vi "analog2digital_wf_array.vi"(8 "error in (no error)":errorcluster, 11 "analog waveform":waveform(dbl)) -> (0 "error out":errorcluster, 1 "full-scale range (out)":dbl, 2 "resolution (out)":i32=16, 3 "digital array":digitalwaveform[](array[waveform]))   [LabVIEW 2015]
uses:
  <vilib>/Waveform/DWDTOps.llb/DWDT Analog to Digital.vi
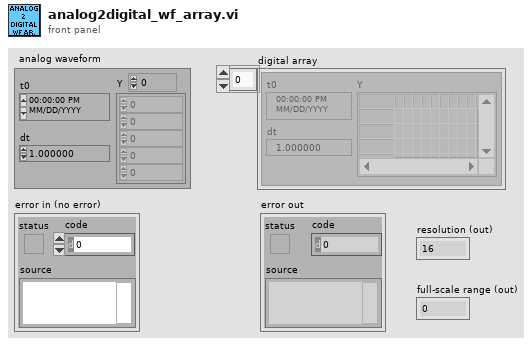
[diagram p1: front panel]
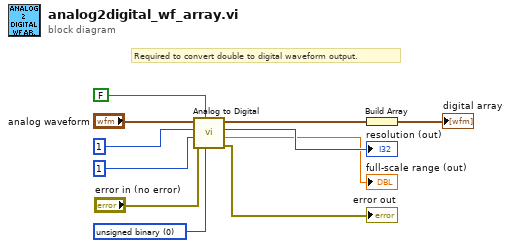
[diagram p0: block diagram]
diagram:
  w6 = u16 0 items=["unsigned binary", "offset binary", "2's complement"] ("data format (offset binary)")
  # "Required to convert double to digital waveform output."
  n1 = call-poly <vilib>:"Analog to Digital.vi"("data format (offset binary)"=w6, "compress digital (T)"=FALSE, "error in (no error)"="error in (no error)", "full-scale range (pk-pk)"=1 ("resolution (16 bit)"), "resolution (16 bit)"=1, "analog waveform"="analog waveform") -> ("error out"=→"error out":errorcluster, "full-scale range (out)"=→"full-scale range (out)":dbl, "resolution (out)"=→"resolution (out)":i32, "digital waveform"=w10:digitalwaveform)  [unwired: 2 in]
  n2 = Build Array(w10) -> (→"digital array":digitalwaveform[])
